vi "Stop Process.vi"(0 "Stop / Start Reactor X":refnum<vi>, 1 "System Idle Pressure X":refnum<vi>, 2 "Reactor Number":i32, 3 "Logging Data X":refnum<vi>, 4 "Countdown X":refnum<vi>, 5 "Save File Connection X":refnum<vi>, 6 "Save File JSON Connection X":refnum<vi>, 7 "Header Connection txt X":refnum<vi>, 8 "Valves on Shared 1":i32, 9 "Stop Program":refnum<vi>, 10 "Valves on Shared 2":i32, 11 "Queue System":refnum<vi>, 12 "Number of Reactors":i32, 13 "System JSON Queue":refnum<vi>, 14 "Valves Per Reactor":i32, 15 "Current Locks":refnum<vi>, 16 "Pump Valves":i32[](array[numeric]), 17 "Current Valve State X":refnum<vi>, 18 "Reactor Name":string="Lock Request:", 19 "Debug Mode X":refnum<vi>, 20 "Wait Before Start (s) X":refnum<vi>, 21 "Number of Shared Lines":i32, 22 "Start Time Reactor X":refnum<vi>, 24 "Reactor Selector":T1(ring), 25 "Time Elapsed X":refnum<vi>, 27 "GUID X":refnum<vi>) -> ()   [LabVIEW 2021]
uses:
  <vilib>/Utility/error.llb/DialogType.ctl
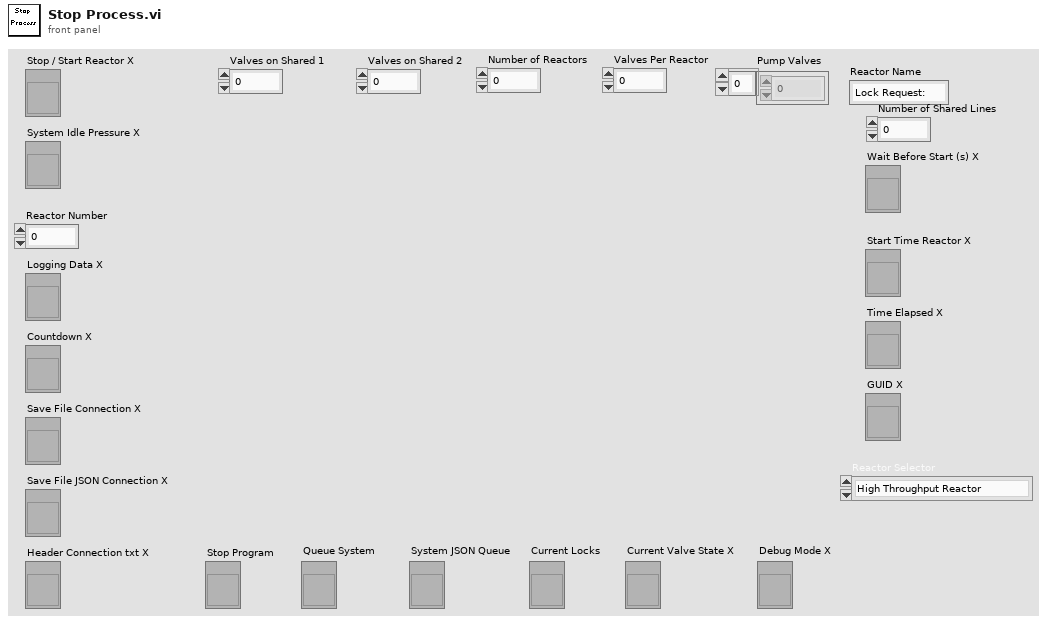
[diagram p1: front panel]
types:
  T1 = enum16{"High Throughput Reactor", "In Situ Reactor", "MLD Reactor"}
  T2 = enum16{"Lock", "Release", "Check", "Check All", "Release All"}
  T3 = cluster{"type":string, "meta":string, "payload":cluster{"TimeElapsed":string, "GUID":string, "EndTime":string}}
  T4 = cluster{"TimeElapsed":string, "GUID":string, "EndTime":string}
  T5 = typedef "DialogType.ctl" = u16
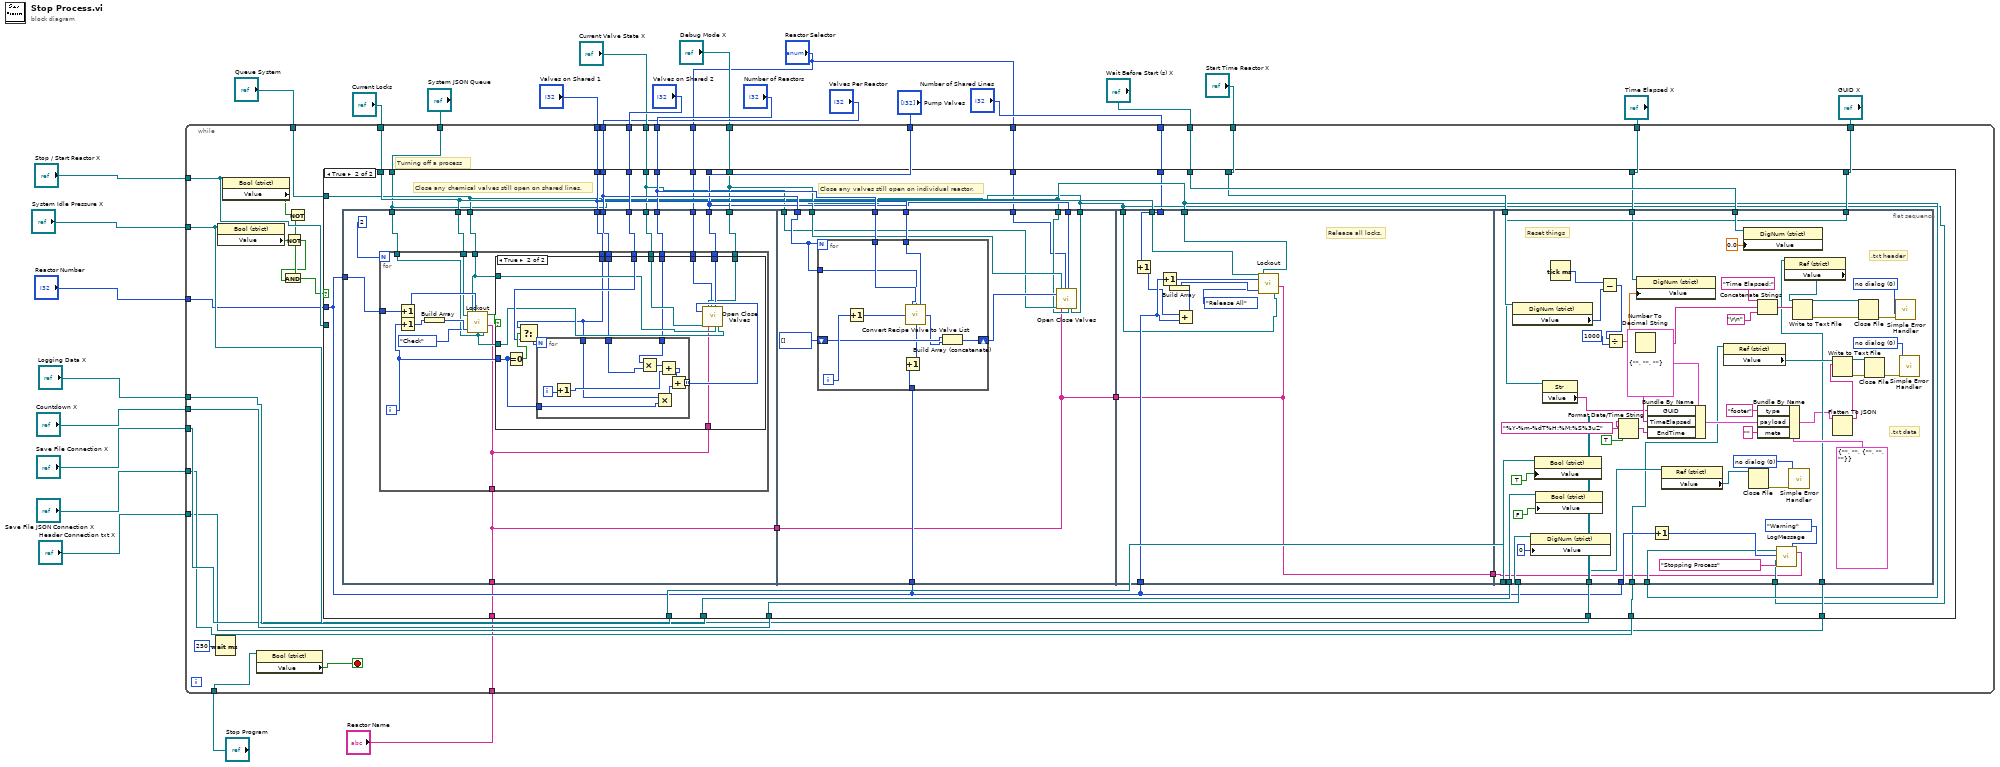
[diagram p0: block diagram]
diagram:
  n1 = while {
    tunnel: "Stop / Start Reactor X" -> [w60]
    tunnel: "System Idle Pressure X" -> [w59]
    tunnel: "Reactor Number" -> [w58]
    tunnel: "Logging Data X" -> [w57]
    tunnel: "Countdown X" -> [w55]
    tunnel: "Save File Connection X" -> [w54]
    tunnel: "Wait Before Start (s) X" -> [w53]
    tunnel: "Save File JSON Connection X" -> [w52]
    tunnel: "Start Time Reactor X" -> [w51]
    tunnel: "Time Elapsed X" -> [w50]
    tunnel: "Header Connection txt X" -> [w49]
    tunnel: "GUID X" -> [w48]
    tunnel: "Stop Program" -> [w46]
    tunnel: "Queue System" -> [w45]
    tunnel: "Current Locks" -> [w44]
    tunnel: "System JSON Queue" -> [w43]
    tunnel: "Valves on Shared 1" -> [w42]
    tunnel: "Valves on Shared 2" -> [w41]
    tunnel: "Pump Valves" -> [w40]
    tunnel: "Current Valve State X" -> [w39]
    tunnel: "Number of Reactors" -> [w38]
    tunnel: "Valves Per Reactor" -> [w37]
    tunnel: "Debug Mode X" -> [w36]
    tunnel: "Reactor Name" -> [w30]
    tunnel: "Number of Shared Lines" -> [w29]
    tunnel: "Reactor Selector" -> [w28]
    tunnel: "Reactor Selector" -> [w27]
    stop <- w47 stop-if-true
    # "Turning off a process"
    n2 = Wait (ms)(milliseconds to wait=u32 250 ("millisecond multiple")) -> ()  [unwired: 1 out]
    n3 = property class="Bool (strict)"(reference=w59) -> ("Value"=w35:bool)  [unwired: 1 in, 2 out]
    n4 = property class="Bool (strict)"(reference=w60) -> ("Value"=w34:bool)  [unwired: 1 in, 2 out]
    n5 = property class="Bool (strict)"(reference=w46) -> ("Value"=w47:bool)  [unwired: 1 in, 2 out]
    n6 = Not(x=w35) -> (.not. x?=w31:bool)
    n7 = Not(x=w34) -> (.not. x?=w32:bool)
    n8 = And(x=w32, y=w31) -> (x .and. y?=w33:bool)
    n9 = case shown="True" w33 {
      tunnel: w58 -> [_ w83]
      tunnel: w60 -> [_ _]
      tunnel: w59 -> [_ w88]
      tunnel: w57 -> [_ w87]
      tunnel: w55 -> [_ w86]
      tunnel: w54 -> [_ w85]
      tunnel: w53 -> [_ w84]
      tunnel: w52 -> [_ w82]
      tunnel: w51 -> [_ w81]
      tunnel: w50 -> [_ w80]
      tunnel: w49 -> [_ w79]
      tunnel: w48 -> [_ w78]
      tunnel: w45 -> [_ w69]
      tunnel: w44 -> [_ w70]
      tunnel: w43 -> [_ w68]
      tunnel: w42 -> [_ w74]
      tunnel: w41 -> [_ w77]
      tunnel: w40 -> [_ w72]
      tunnel: w39 -> [_ w71]
      tunnel: w38 -> [_ w75]
      tunnel: w37 -> [_ w76]
      tunnel: w36 -> [_ w73]
      tunnel: w30 -> [_ w67]
      tunnel: w29 -> [_ w63]
      tunnel: w28 -> [_ w62]
      tunnel: w27 -> [_ w61]
      frame False {
        # "If not, do nothing."
      }
      frame True {
        # "Close any valves still open on individual reactor."
        # "Close any chemical valves still open on shared lines."
        n10 = flat-sequence {
          tunnel: w83 -> [w102]
          tunnel: w69 -> [w100]
          tunnel: w70 -> [w99]
          tunnel: w68 -> [w98]
          tunnel: w74 -> [w97]
          tunnel: w77 -> [w96]
          tunnel: w72 -> [w95]
          tunnel: w71 -> [w94]
          tunnel: w75 -> [w93]
          tunnel: w76 -> [w92]
          tunnel: w73 -> [w91]
          tunnel: w67 -> [w90]
          tunnel: [w90] -> w66
          tunnel: w62 -> [w89]
          tunnel: w83 -> [w159]
          tunnel: w76 -> [w155]
          tunnel: w75 -> [w156]
          tunnel: w74 -> [w154]
          tunnel: w73 -> [w153]
          tunnel: w72 -> [w152]
          tunnel: w71 -> [w151]
          tunnel: w69 -> [w150]
          tunnel: w68 -> [w149]
          tunnel: w66 -> [w148]
          tunnel: [w148] -> w65
          tunnel: w61 -> [w147]
          tunnel: w83 -> [w180]
          tunnel: w68 -> [w175]
          tunnel: w69 -> [w174]
          tunnel: w70 -> [w173]
          tunnel: w65 -> [w172]
          tunnel: [w172] -> w64
          tunnel: w63 -> [w171]
          tunnel: w88 -> [w234]
          tunnel: w87 -> [w233]
          tunnel: w86 -> [w232]
          tunnel: w85 -> [w194]
          tunnel: w84 -> [w231]
          tunnel: w83 -> [w223]
          tunnel: w82 -> [w191]
          tunnel: w81 -> [w220]
          tunnel: w80 -> [w203]
          tunnel: w79 -> [w193]
          tunnel: w78 -> [w204]
          tunnel: w69 -> [w183]
          tunnel: w68 -> [w182]
          tunnel: w64 -> [w181]
          frame #0 {
            n11 = for {
              N: 2 -> [_]
              tunnel: w102 -> [w121]
              tunnel: w100 -> [w109]
              tunnel: w99 -> [w114]
              tunnel: w98 -> [w108]
              tunnel: w97 -> [w113]
              tunnel: w96 -> [w112]
              tunnel: w95 -> [w111]
              tunnel: w94 -> [w110]
              tunnel: w93 -> [w107]
              tunnel: w92 -> [w106]
              tunnel: w91 -> [w105]
              tunnel: w90 -> [w104]
              tunnel: w89 -> [w103]
              i -> [w119]
              n12 = Increment(x=w121) -> (x+1=w117:i32)
              n13 = Increment(x=w119) -> (x+1=w120:i32)
              n14 = Build Array(w120) -> (w116:i32[])
              n15 = call "Lockout.vi"("Locks"=w114, "ID"=w117, "Queue System"=w109, "Request Type"=enum16{"Lock", "Release", "Check"}."Check", "Request Array"=w116, "Reactor Name"=w104, "JSON Queue"=w108) -> ("Response"=w118:bool)  [unwired: 1 out]
              n16 = case shown="True" w118 {
                tunnel: w119 -> [_ w134]
                tunnel: w113 -> [_ w125]
                tunnel: w112 -> [_ w132]
                tunnel: w111 -> [_ w131]
                tunnel: w110 -> [_ w130]
                tunnel: w109 -> [_ w129]
                tunnel: w108 -> [_ w128]
                tunnel: w107 -> [_ w127]
                tunnel: w106 -> [_ w126]
                tunnel: w105 -> [_ w124]
                tunnel: w104 -> [_ w123]
                tunnel: w103 -> [_ w122]
                frame False {
                }
                frame True {
                  n17 = Equal To 0?(x=w134) -> (x = 0?=w135:bool)
                  n18 = Select(t=w125, s=w135, f=w132) -> (s? t:f=w136:i32)
                  n19 = for {
                    N: w136 -> [_]
                    tunnel: w134 -> [w145]
                    tunnel: [w140] -> w133 mode=indexing
                    tunnel: w127 -> [w139]
                    tunnel: w126 -> [w138]
                    tunnel: w125 -> [w137]
                    i -> [w146]
                    n20 = Increment(x=w146) -> (x+1=w143:i32)
                    n21 = Multiply(x=w139, y=w138) -> (x*y=w144:i32)
                    n22 = Multiply(x=w137, y=w145) -> (x*y=w141:i32)
                    n23 = Add(x=w144, y=w143) -> (x+y=w142:i32)
                    n24 = Add(x=w142, y=w141) -> (x+y=w140:i32)
                  }
                  n25 = call "Open Close Valves.vi"("Valves to Close"=w133, "Current Valve State"=w130, "Debug Mode"=w124, "Reactor Name"=w123, "Reactor Selector"=w122, "Pump Valves"=w131, "System Queue"=w129, "JSON Queue"=w128) -> ()  [unwired: 12 in]
                }
              }
            }
          }
          frame #1 {
            n26 = for {
              N: w155 -> [_]
              tunnel: w159 -> [w167]
              shift-right: [w166] -> w157
              shift-left: i32[] [] -> [w165]
              tunnel: w156 -> [w162]
              tunnel: w155 -> [w161]
              tunnel: w154 -> [w160]
              i -> [w169]
              n27 = Increment(x=w169) -> (x+1=w168:i32)
              n28 = Increment(x=w167) -> (x+1=w163:i32)
              n29 = call "Convert Recipe Valve to Valve List.vi"("Valves on Shared Lines"=w160, "Valves Per Reactor"=w161, "Number of Reactors"=w162, "Reactor ID#"=w163, "Valve Number"=w168) -> ("Valve List"=w164:i32[])  [unwired: 10 in]
              n30 = Build Array (concatenate)(w165, w164) -> (w166:i32[])
            }
            n31 = call "Open Close Valves.vi"("Valves to Close"=w157, "Current Valve State"=w151, "Debug Mode"=w153, "Reactor Name"=w148, "Reactor Selector"=w147, "Pump Valves"=w152, "System Queue"=w150, "JSON Queue"=w149) -> ()  [unwired: 12 in]
          }
          frame #2 {
            # "Release all locks."
            n32 = Increment(x=w171) -> (x+1=w170:i32)
            n33 = Increment(x=w180) -> (x+1=w178:i32)
            n34 = Add(x=w170, y=w180) -> (x+y=w179:i32)
            n35 = Build Array(w179) -> (w177:i32[])
            n36 = call "Lockout.vi"("Locks"=w173, "ID"=w178, "Queue System"=w174, "Request Type"=T2."Release All", "Request Array"=w177, "Reactor Name"=w172, "JSON Queue"=w175) -> ()  [unwired: 2 out]
          }
          frame #3 {
            w207 = T5 0 items=["no dialog", "OK message", "continue or stop message", "OK message + warnings", "continue/stop + warnings"] ("type of dialog (OK msg:1)")
            w208 = T5 0 items=["no dialog", "OK message", "continue or stop message", "OK message + warnings", "continue/stop + warnings"] ("type of dialog (OK msg:1)")
            w225 = T5 0 items=["no dialog", "OK message", "continue or stop message", "OK message + warnings", "continue/stop + warnings"] ("type of dialog (OK msg:1)")
            # ".txt data"
            # ".txt header"
            # "Reset things"
            n37 = property class="DigNum (strict)"(reference=w220) -> ("Value"=w221:i32)  [unwired: 1 in, 2 out]
            n38 = property class="DigNum (strict)"(reference=w232, "Value"=0) -> ()  [unwired: 1 in, 2 out]
            n39 = property class="Bool (strict)"(reference=w234, "Value"=TRUE) -> ()  [unwired: 1 in, 2 out]
            n40 = property class="Bool (strict)"(reference=w233, "Value"=FALSE) -> ()  [unwired: 1 in, 2 out]
            n41 = property class="Str"(reference=w204) -> ("Value"=w205:string)  [unwired: 1 in, 2 out]
            n42 = Tick Count (ms)() -> (millisecond timer value=w222:u32)
            n43 = Subtract(x=w222, y=w221) -> (x-y=w202:u32)
            n44 = Divide(x=w202, y=u32 1000) -> (x/y=w200:dbl)
            n45 = Format Date/Time String(time format string (%c)="%Y-%m-%dT%H:%M:%S%3uZ", UTC format=TRUE) -> (date/time string=w196:string)  [unwired: 1 in]
            n46 = Number To Decimal String(number=w200) -> (decimal integer string=w209:string)  [unwired: 1 in]
            n47 = property class="DigNum (strict)"(reference=w203, "Value"=w200) -> ()  [unwired: 1 in, 2 out]
            n48 = Bundle By Name(cluster=T4 {"TimeElapsed"="", "GUID"="", "EndTime"=""} ("input cluster"), "GUID"=w205, "TimeElapsed"=w209, "EndTime"=w196) -> (w192:T4)
            n49 = Increment(x=w223) -> (x+1=w187:i32)
            n50 = property class="Ref (strict)"(reference=w194) -> ("Value"=w227:refnum<file>)  [unwired: 1 in, 2 out]
            n51 = property class="Ref (strict)"(reference=w191) -> ("Value"=w197:refnum<file>)  [unwired: 1 in, 2 out]
            n52 = property class="DigNum (strict)"(reference=w231, "Value"=sgl 0.0) -> ()  [unwired: 1 in, 2 out]
            n53 = Close File(refnum=w227) -> (error out=w226:errorcluster)  [unwired: 1 in, 1 out]
            n54 = Concatenate Strings("Time Elapsed:" ("string"), w209, "\r\n") -> (w218:string)
            n55 = Bundle By Name(cluster=T3 {"type"="", "meta"="", "payload"={"TimeElapsed"="", "GUID"="", "EndTime"=""}} ("input cluster"), "type"="footer", "payload"=w192, "meta"="") -> (w185:T3)
            n56 = call "LogMessage.vi"("Type"=enum16{"Locks", "Warning"}."Warning", "Reactor Name"=w181, "Log Entry"="Stopping Process", "System JSON Queue"=w182, "ID Number"=w187, "System Queue"=w183) -> ()
            n57 = property class="Ref (strict)"(reference=w193) -> ("Value"=w206:refnum<file>)  [unwired: 1 in, 2 out]
            n58 = call <vilib>:"Simple Error Handler.vi"("type of dialog (OK msg:1)"=w225, "error in (no error)"=w226) -> ()  [unwired: 3 in, 5 out]
            n59 = Write to Text File(file (use dialog)=w206, text=w218) -> (refnum out=w216:refnum<file>, error out=w217:errorcluster)  [unwired: 2 in, 1 out]
            n60 = Flatten To JSON(anything=w185) -> (JSON string=w184:string)  [unwired: 2 in, 1 out]
            n61 = Write to Text File(file (use dialog)=w197, text=w184) -> (refnum out=w211:refnum<file>, error out=w212:errorcluster)  [unwired: 2 in, 1 out]
            n62 = Close File(refnum=w216, error in=w217) -> (error out=w214:errorcluster)  [unwired: 1 out]
            n63 = Close File(refnum=w211, error in=w212) -> (error out=w210:errorcluster)  [unwired: 1 out]
            n64 = call <vilib>:"Simple Error Handler.vi"("type of dialog (OK msg:1)"=w208, "error in (no error)"=w214) -> ()  [unwired: 3 in, 5 out]
            n65 = call <vilib>:"Simple Error Handler.vi"("type of dialog (OK msg:1)"=w207, "error in (no error)"=w210) -> ()  [unwired: 3 in, 5 out]
          }
        }
      }
    }
  }
